vi "Find And Replace Pattern.vi"(2 "Ignore Case? (false)":bool, 3 "Replace All? (false)":bool, 4 "Offset (0)":i32, 5 "Replace Pattern (\"\")":string, 6 "Search Pattern":string, 7 "String in":string) -> (0 "Offset Past Replacement":i32, 1 "String out":string)   [LabVIEW 2017]
doc: "Searches for a Regular Expression and replaces it with the given pattern.\n\n<B>Search Pattern</B> - The Regular Expression pattern to search for.\n<B>Replace Pattern</B> - The pattern to replace Search Pattern with. Parenthesized items in <B>Search Pattern</B> can be referenced with $n where n is the index of the parenthesized item. Dollar signs ($) can be explicitly put in by prefixing them with a backslash (\\), for example \\$5 would be $5 and $5 would represent the 5th parenthesized item.\n<B>String in</B> - The string to modify.\n<B>Offset</B> - The offset in <B>String in</B> to start modifying.\n<B>Ignore Case?</B> - Determines if case will matter in <B>Search Pattern</B>.\n<B>Replace All?</B> - If true, all instances of <B>Search Pattern</B> in <B>String in</B> will be replaced with <B>Replace Pattern</B>, otherwise just the first instance will be changed.\n<B>Offset Past Replacement</B> - The offset of the first character after the last replacement done.\n<B>String out</B> - The modified string with <B>Search Pattern</B> replaced with <B>Replace Pattern</B>."
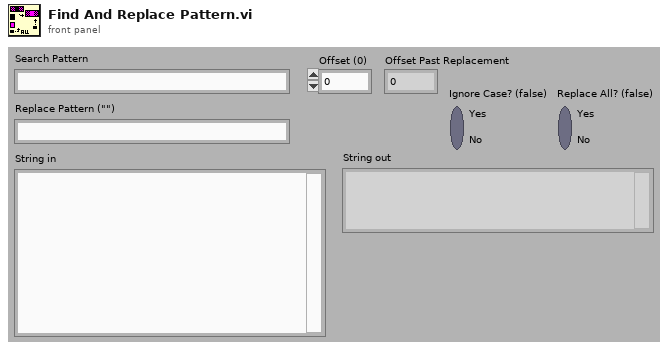
[diagram p1: front panel]
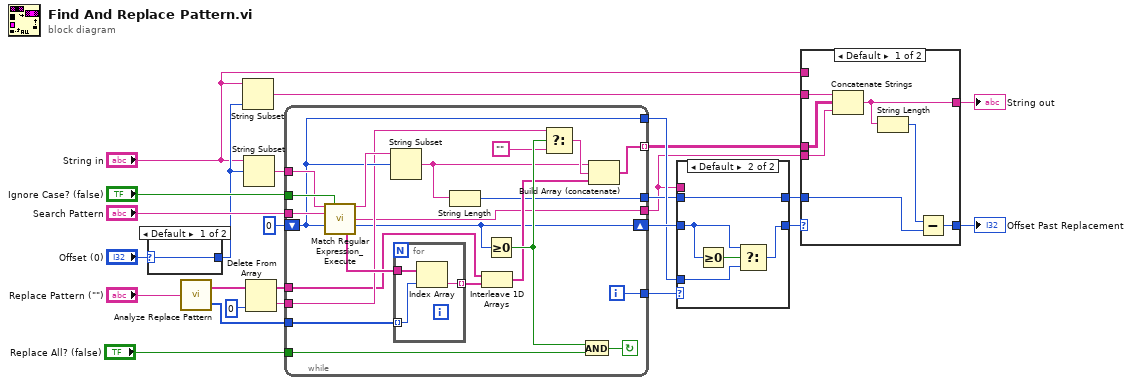
[diagram p0: block diagram]
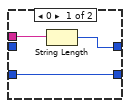
[diagram p4: hidden frame]
diagram:
  n1 = case shown="Default" "Offset (0)" {
    selector: "Offset (0)" -> [w26 _]
    tunnel: [w26 _] -> w12
    frame Default {
    }
    frame ..0 {
    }
  }
  n2 = call <vilib>:"Analyze Replace Pattern.vi"("Replace Pattern"="Replace Pattern (\"\")") -> ("Replace Constants"=w10:string[], "Replace Variable Indexes"=w21:i32[])
  n3 = String Subset(string="String in", length (rest)=w12) -> (substring=w7:string)  [unwired: 1 in]
  n4 = String Subset(string="String in", offset (0)=w12) -> (substring=w17:string)  [unwired: 1 in]
  n5 = Delete From Array(array=w10, index=0) -> (deleted portion=w8:string, array with subset deleted=w9:string[])  [unwired: 1 in]
  n6 = while {
    tunnel: "Search Pattern" -> [w48]
    shift-right: [w31] -> w19
    shift-left: 0 ("whole match offset") -> [w36]
    tunnel: "Ignore Case? (false)" -> [w47]
    tunnel: w21 -> [w44]
    tunnel: w17 -> [w45]
    tunnel: "Replace All? (false)" -> [w42]
    tunnel: [w37] -> w20
    tunnel: [w36] -> w18
    tunnel: w9 -> [w33]
    tunnel: w8 -> [w35]
    tunnel: [w29] -> w4
    tunnel: [w28] -> w6 mode=indexing
    tunnel: [w27] -> w2
    i -> [w37]
    stop <- w41 continue-if-true
    n7 = call <vilib>:"Match Regular Expression_Execute.vi"("input string"=w45, "ignore case? (F)"=w47, "regular expression"=w48, "offset (0)"=w36) -> ("before match"=w46:string, "after match"=w27:string, "whole match offset"=w31:i32, "matched substrings"=w43:string[])  [unwired: 6 in, 2 out]
    n8 = String Subset(string=w46, offset (0)=w36) -> (substring=w30:string)  [unwired: 1 in]
    n9 = for {
      tunnel: w44 -> [w50] mode=indexing
      tunnel: w43 -> [w51]
      tunnel: [w49] -> w34 mode=indexing
      n10 = Index Array(array=w51, index=w50) -> (element=w49:string)
    }
    n11 = String Length(string=w30) -> (length=w29:i32)
    n12 = Interleave 1D Arrays(w33, w34) -> (w32:string[])
    n13 = Greater Or Equal To 0?(x=w31) -> (x >= 0?=w39:bool)
    n14 = Select(t=w35, s=w39, f="") -> (s? t:f=w40:string)
    n15 = And(x=w39, y=w42) -> (x .and. y?=w41:bool)
    n16 = Build Array (concatenate)(w30, w40, w32) -> (w28:string[])
  }
  n17 = case shown="Default" w20 {
    tunnel: w19 -> [w54 w57]
    tunnel: [w54 w58] -> w15
    tunnel: w18 -> [_ w56]
    tunnel: w4 -> [_ w55]
    tunnel: [w52 w55] -> w3
    tunnel: w2 -> [w53 _]
    frame 0 {
      n18 = String Length(string=w53) -> (length=w52:i32)
    }
    frame Default {
      n19 = Greater Or Equal To 0?(x=w57) -> (x >= 0?=w59:bool)
      n20 = Select(t=w57, s=w59, f=w56) -> (s? t:f=w58:i32)
    }
  }
  n21 = case shown="Default" w15 {
    selector: w15 -> [_ w68]
    tunnel: [w64 w68] -> w14
    tunnel: [w60 w67] -> w1
    tunnel: w3 -> [w65 _]
    tunnel: w7 -> [w63 _]
    tunnel: w6 -> [w62 _]
    tunnel: w2 -> [w61 _]
    tunnel: "String in" -> [_ w67]
    frame Default {
      n22 = Concatenate Strings(w63, w62, w61) -> (w60:string)
      n23 = String Length(string=w60) -> (length=w66:i32)
      n24 = Subtract(x=w66, y=w65) -> (x-y=w64:i32)
    }
    frame -1 {
    }
  }
  "String out" <- w1
  "Offset Past Replacement" <- w14
